vi "Test Simple Server.vi"() -> ()   [LabVIEW 2020]
uses:
  source/PV Data/NT Base/NT Base.lvclass
  source/Server/Server/Server.lvclass
  source/Server/Server/Fetch - U64.vi
  source/Server/Server/Fetch - U16.vi
  source/Server/Server/Post - I16.vi
  source/Server/Server/Post - U16.vi
  source/Server/Server/Fetch - U32.vi
  source/Server/Server/Post - I8.vi
  source/Server/Server/Post - U32.vi
  source/Server/Server/Post - U8.vi
  source/Server/Server/Post - U64.vi
  source/Server/Server/Post - I64.vi
  source/Server/Server/Fetch - I64.vi
  source/Server/Server/Fetch - I8.vi
  source/Server/Server/Add PV - Any Class.vi
  source/Server/Server/Fetch - I16.vi
  source/Server/Server/Fetch - I32.vi
  source/Server/Server/Fetch - U8.vi
  source/Server/Server/Post - I32.vi
panel:
  in  "U64":u64
  in  "U32":u32
  in  "U16":u16
  in  "U8":u8
  in  "I64":i64
  in  "I32":i32
  in  "I16":i16
  in  "I8":i8
  in  "stop":bool
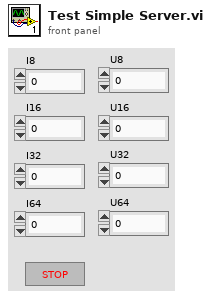
[diagram p1: front panel]
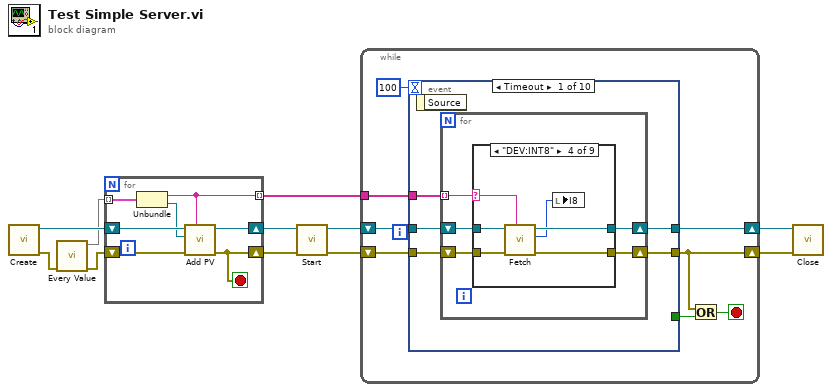
[diagram p0: block diagram]
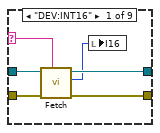
[diagram p2: hidden frame]
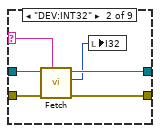
[diagram p3: hidden frame]
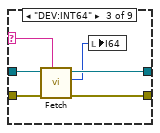
[diagram p4: hidden frame]
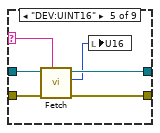
[diagram p5: hidden frame]
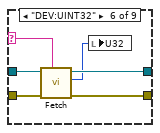
[diagram p6: hidden frame]
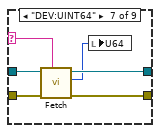
[diagram p7: hidden frame]
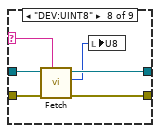
[diagram p8: hidden frame]
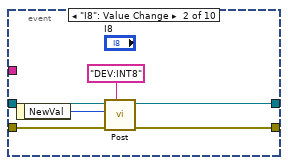
[diagram p10: hidden frame]
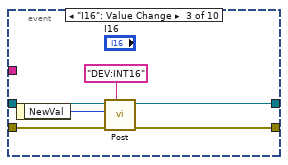
[diagram p11: hidden frame]
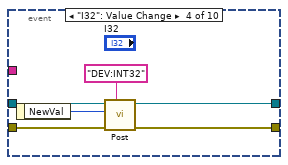
[diagram p12: hidden frame]
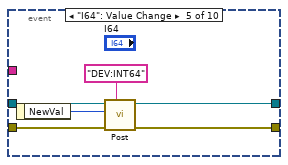
[diagram p13: hidden frame]
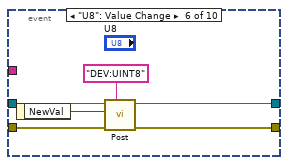
[diagram p14: hidden frame]
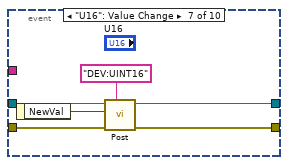
[diagram p15: hidden frame]
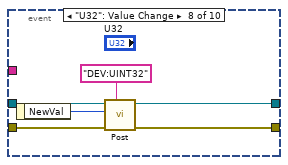
[diagram p16: hidden frame]
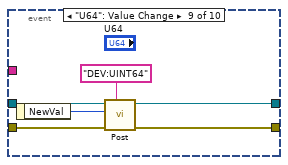
[diagram p17: hidden frame]
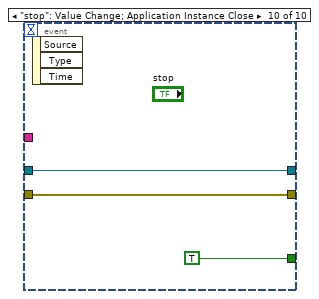
[diagram p18: hidden frame]
diagram:
  n1 = call "Create.vi"() -> ("error out"=w11:errorcluster, "Server out"=w10:refnum<class "Server.lvclass">)  [unwired: 10 in]
  n2 = call "Every Value.vi"("error in (no error)"=w11) -> ("error out"=w9:errorcluster, "values"=w8:map{string, refnum<class "NT Base.lvclass">})  [unwired: 9 in]
  n3 = for {
    shift-right: [w18] -> w6
    shift-left: w10 -> [w16]
    tunnel: [w13] -> w3 mode=indexing
    shift-right: [w17] -> w7
    shift-left: w9 -> [w15]
    tunnel: w8 -> [w14] mode=indexing
    stop <- w17 stop-if-true
    n4 = Unbundle(w14) -> ("PV name"=w13:string, "PV Data.lvlib:NT Base.lvclass"=w12:refnum<class "NT Base.lvclass">)
    n5 = call-poly "Add PV.vi"("PV name"=w13, "error in (no error)"=w15, "initial value"=w12, "Server in"=w16) -> ("error out"=w17:errorcluster, "Server out"=w18:refnum<class "Server.lvclass">)  [unwired: 5 in, 1 out]
  }
  n6 = call-dynamic "Start.vi"("error in (no error)"=w7, "Server in"=w6) -> ("error out"=w5:errorcluster, "Server out"=w4:refnum<class "Server.lvclass">)  [unwired: 8 in]
  n7 = while {
    shift-right: [w21] -> w2
    shift-left: w5 -> [w26]
    shift-right: [w24] -> w1
    shift-left: w4 -> [w25]
    tunnel: w3 -> [w19]
    stop <- w23 stop-if-true
    n8 = event shown="[0] Timeout" {
      selector: _ -> [_ _ _ _ _ _ _ _ _ _]
      dyn-events: _ -> [_ _ _ _ _ _ _ _ _ _]
      timeout: 100 -> [_ _ _ _ _ _ _ _ _ _]
      tunnel: [w27 w88 w94 w100 w106 w112 w118 w124 w130 w137] -> w21
      tunnel: w26 -> [w29 w91 w97 w103 w109 w115 w121 w127 w133 w137]
      tunnel: w25 -> [w30 w90 w96 w102 w108 w114 w120 w126 w132 w136]
      tunnel: [w28 w89 w95 w101 w107 w113 w119 w125 w131 w136] -> w24
      tunnel: [_ _ _ _ _ _ _ _ _ TRUE] -> w22
      tunnel: w19 -> [w31 _ _ _ _ _ _ _ _ _]
      event Timeout {
        n9 = event-data() -> ()  [unwired: 1 in, 1 out]
        n10 = for {
          tunnel: w31 -> [w36] mode=indexing
          shift-right: [w33] -> w28
          shift-left: w30 -> [w35]
          shift-right: [w32] -> w27
          shift-left: w29 -> [w34]
          n11 = case shown="\"DEV:INT8\"" w36 {
            selector: w36 -> [w39 w45 w51 w57 w63 w69 w75 w81 _]
            tunnel: w35 -> [w41 w47 w53 w59 w65 w71 w77 w83 w86]
            tunnel: w34 -> [w42 w48 w54 w60 w66 w72 w78 w84 w85]
            tunnel: [w40 w46 w52 w58 w64 w70 w76 w82 w85] -> w32
            tunnel: [w38 w44 w50 w56 w62 w68 w74 w80 w86] -> w33
            frame "DEV:INT16" {
              n12 = call-poly "Fetch.vi"("PV name"=w39, "error in"=w42, "Server in"=w41) -> ("error out"=w40:errorcluster, "value"=w37:i16, "Server out"=w38:refnum<class "Server.lvclass">)  [unwired: 4 in, 2 out]
              n13 = local write "I16"(w37) -> ()
            }
            frame "DEV:INT32" {
              n14 = call-poly "Fetch.vi"("PV name"=w45, "error in"=w48, "Server in"=w47) -> ("error out"=w46:errorcluster, "value"=w43:i32, "Server out"=w44:refnum<class "Server.lvclass">)  [unwired: 4 in, 2 out]
              n15 = local write "I32"(w43) -> ()
            }
            frame "DEV:INT64" {
              n16 = call-poly "Fetch.vi"("PV name"=w51, "error in"=w54, "Server in"=w53) -> ("error out"=w52:errorcluster, "value"=w49:i64, "Server out"=w50:refnum<class "Server.lvclass">)  [unwired: 4 in, 2 out]
              n17 = local write "I64"(w49) -> ()
            }
            frame "DEV:INT8" {
              n18 = call-poly "Fetch.vi"("PV name"=w57, "error in"=w60, "Server in"=w59) -> ("error out"=w58:errorcluster, "value"=w55:i8, "Server out"=w56:refnum<class "Server.lvclass">)  [unwired: 4 in, 2 out]
              n19 = local write "I8"(w55) -> ()
            }
            frame "DEV:UINT16" {
              n20 = call-poly "Fetch.vi"("PV name"=w63, "error in"=w66, "Server in"=w65) -> ("error out"=w64:errorcluster, "value"=w61:u16, "Server out"=w62:refnum<class "Server.lvclass">)  [unwired: 4 in, 2 out]
              n21 = local write "U16"(w61) -> ()
            }
            frame "DEV:UINT32" {
              n22 = call-poly "Fetch.vi"("PV name"=w69, "error in"=w72, "Server in"=w71) -> ("error out"=w70:errorcluster, "value"=w67:u32, "Server out"=w68:refnum<class "Server.lvclass">)  [unwired: 4 in, 2 out]
              n23 = local write "U32"(w67) -> ()
            }
            frame "DEV:UINT64" {
              n24 = call-poly "Fetch.vi"("PV name"=w75, "error in"=w78, "Server in"=w77) -> ("error out"=w76:errorcluster, "value"=w73:u64, "Server out"=w74:refnum<class "Server.lvclass">)  [unwired: 4 in, 2 out]
              n25 = local write "U64"(w73) -> ()
            }
            frame "DEV:UINT8" {
              n26 = call-poly "Fetch.vi"("PV name"=w81, "error in"=w84, "Server in"=w83) -> ("error out"=w82:errorcluster, "value"=w79:u8, "Server out"=w80:refnum<class "Server.lvclass">)  [unwired: 4 in, 2 out]
              n27 = local write "U8"(w79) -> ()
            }
            frame Default {
            }
          }
        }
      }
      event "I8": Value Change {
        n28 = event-data() -> ("NewVal"=w92:i8)  [unwired: 1 in]
        n29 = call-poly "Post.vi"("PV name"="DEV:INT8", "error in (no error)"=w91, "value"=w92, "Server in"=w90) -> ("error out"=w88:errorcluster, "Server out"=w89:refnum<class "Server.lvclass">)  [unwired: 6 in]
      }
      event "I16": Value Change {
        n30 = event-data() -> ("NewVal"=w98:i16)  [unwired: 1 in]
        n31 = call-poly "Post.vi"("PV name"="DEV:INT16", "error in (no error)"=w97, "value"=w98, "Server in"=w96) -> ("error out"=w94:errorcluster, "Server out"=w95:refnum<class "Server.lvclass">)  [unwired: 6 in]
      }
      event "I32": Value Change {
        n32 = event-data() -> ("NewVal"=w104:i32)  [unwired: 1 in]
        n33 = call-poly "Post.vi"("PV name"="DEV:INT32", "error in (no error)"=w103, "value"=w104, "Server in"=w102) -> ("error out"=w100:errorcluster, "Server out"=w101:refnum<class "Server.lvclass">)  [unwired: 6 in]
      }
      event "I64": Value Change {
        n34 = event-data() -> ("NewVal"=w110:i64)  [unwired: 1 in]
        n35 = call-poly "Post.vi"("PV name"="DEV:INT64", "error in (no error)"=w109, "value"=w110, "Server in"=w108) -> ("error out"=w106:errorcluster, "Server out"=w107:refnum<class "Server.lvclass">)  [unwired: 6 in]
      }
      event "U8": Value Change {
        n36 = event-data() -> ("NewVal"=w116:u8)  [unwired: 1 in]
        n37 = call-poly "Post.vi"("PV name"="DEV:UINT8", "error in (no error)"=w115, "value"=w116, "Server in"=w114) -> ("error out"=w112:errorcluster, "Server out"=w113:refnum<class "Server.lvclass">)  [unwired: 6 in]
      }
      event "U16": Value Change {
        n38 = event-data() -> ("NewVal"=w122:u16)  [unwired: 1 in]
        n39 = call-poly "Post.vi"("PV name"="DEV:UINT16", "error in (no error)"=w121, "value"=w122, "Server in"=w120) -> ("error out"=w118:errorcluster, "Server out"=w119:refnum<class "Server.lvclass">)  [unwired: 6 in]
      }
      event "U32": Value Change {
        n40 = event-data() -> ("NewVal"=w128:u32)  [unwired: 1 in]
        n41 = call-poly "Post.vi"("PV name"="DEV:UINT32", "error in (no error)"=w127, "value"=w128, "Server in"=w126) -> ("error out"=w124:errorcluster, "Server out"=w125:refnum<class "Server.lvclass">)  [unwired: 6 in]
      }
      event "U64": Value Change {
        n42 = event-data() -> ("NewVal"=w134:u64)  [unwired: 1 in]
        n43 = call-poly "Post.vi"("PV name"="DEV:UINT64", "error in (no error)"=w133, "value"=w134, "Server in"=w132) -> ("error out"=w130:errorcluster, "Server out"=w131:refnum<class "Server.lvclass">)  [unwired: 6 in]
      }
      event "stop": Value Change; Application Instance Close {
        n44 = event-data() -> ()  [unwired: 1 in, 3 out]
      }
    }
    n45 = Or(x=w21, y=w22) -> (x .or. y?=w23:bool)
  }
  n46 = call-dynamic "Close.vi"("error in"=w2, "Server in"=w1) -> ()  [unwired: 9 in, 1 out]
